vi "Cell12_PS_Control_Remote.vi"() -> ()   [LabVIEW 2021]
panel:
  in  "Slew Rate":dbl=1.0 format="%#_4g"
  out "error out 3":errorcluster
  in  "Setpoint [T]":dbl format="%#_4g"
  in  "stop":bool
  in  "port":u16=3376
  in  "error in (no error) 2":errorcluster
  in  "Data mac ip address":string="146.201.214.247"
  out "Field [T]":dbl=-17.9883723 format="%#_4g"
  # "[T/min]"
  # "Note\n(1) Exception of the firewall should be configured.\n(2) With some (not all) connection with PC's, it is successful only when the VI is first executed. If the VI is stopped (normally or by aborting), \nthe subsequent connection is only possible with a new port number."
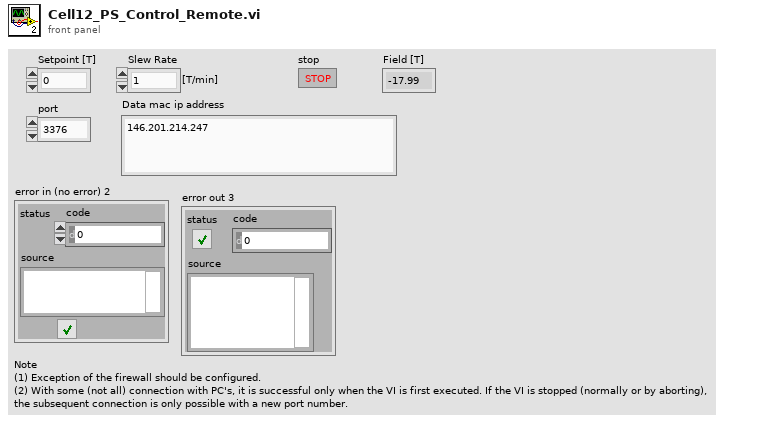
[diagram p1: front panel]
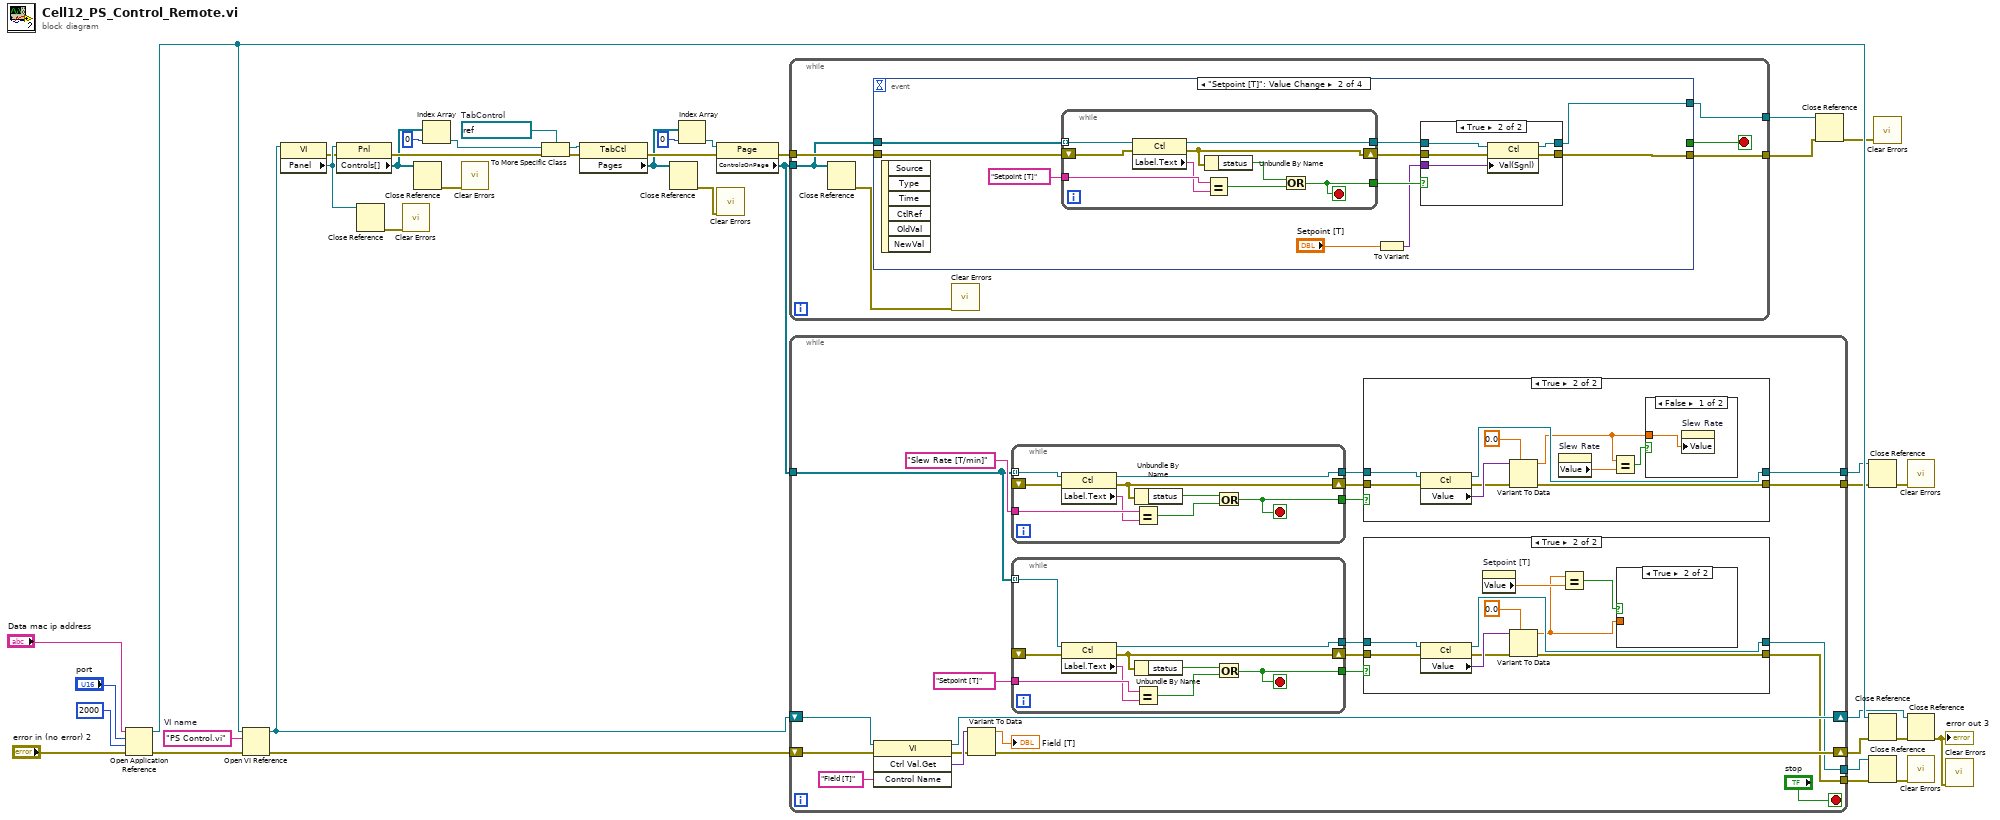
[diagram p0: block diagram]
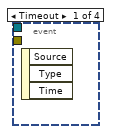
[diagram p2: hidden frame]
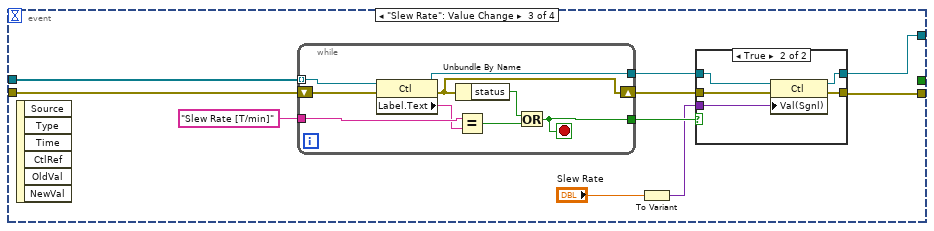
[diagram p4: hidden frame]
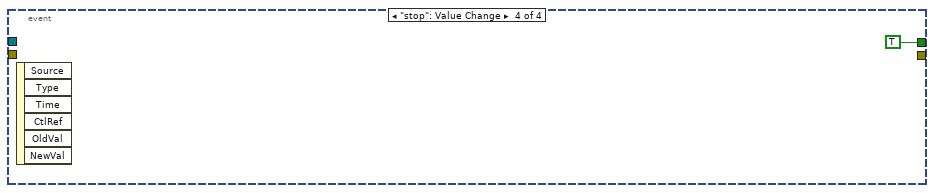
[diagram p6: hidden frame]
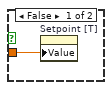
[diagram p8: hidden frame]
diagram:
  w13 = refnum<vi> refnum  # TabControl
  w32 = "PS Control.vi"  # VI name
  n1 = Open Application Reference(8:"error in (no error) 2", 9:2000 ("timeout ms (60000)"), 10:"port", 11:"Data mac ip address") -> (0:w39:errorcluster, 3:w34:refnum<vi>)
  n2 = Open VI Reference(application reference (local)=w34, vi path=w32, error in (no error)=w39) -> (vi reference=w29:refnum<vi>, error out=w28:errorcluster)  [unwired: 3 in]
  n3 = property class="VI"(reference=w29) -> (error out=w16:errorcluster, "Panel"=w19:refnum<vi>)  [unwired: 1 in, 1 out]
  n4 = property class="Pnl"(reference=w19, error in=w16) -> (error out=w25:errorcluster, "Controls[]"=w21:refnum<vi>[])  [unwired: 1 out]
  n5 = Close Reference(reference=w19) -> (error out=w15:errorcluster)  [unwired: 1 in]
  n6 = call <vilib>:"Clear Errors.vi"("error in (no error)"=w15) -> ()  [unwired: 5 in, 2 out]
  n7 = Close Reference(reference=w21) -> (error out=w20:errorcluster)  [unwired: 1 in]
  n8 = Index Array(array=w21, index=0) -> (element=w17:refnum<vi>)
  n9 = call <vilib>:"Clear Errors.vi"("error in (no error)"=w20) -> ()  [unwired: 5 in, 2 out]
  n10 = To More Specific Class(target class=w13, reference=w17, error in=w25) -> (specific class reference=w18:refnum<vi>, error out=w26:errorcluster)
  n11 = property class="TabCtl"(reference=w18, error in=w26) -> (error out=w27:errorcluster, "Pages"=w23:refnum<vi>[])  [unwired: 1 out]
  n12 = Close Reference(reference=w23) -> (error out=w22:errorcluster)  [unwired: 1 in]
  n13 = Index Array(array=w23, index=0) -> (element=w24:refnum<vi>)
  n14 = property class="Page"(reference=w24, error in=w27) -> (error out=w11:errorcluster, "ControlsOnPage"=w10:refnum<vi>[])  [unwired: 1 out]
  n15 = call <vilib>:"Clear Errors.vi"("error in (no error)"=w22) -> ()  [unwired: 5 in, 2 out]
  n16 = while {
    tunnel: w11 -> [w44]
    tunnel: w10 -> [w43]
    tunnel: [w42] -> w2
    tunnel: [w41] -> w1
    stop <- w46 stop-if-true
    n17 = Close Reference(reference=w43) -> (error out=w45:errorcluster)  [unwired: 1 in]
    n18 = event shown="[1] \"Setpoint [T]\": Value Change" {
      selector: _ -> [_ _ _ _]
      dyn-events: _ -> [_ _ _ _]
      timeout: _ -> [_ _ _ _]
      tunnel: [_ _ _ TRUE] -> w46
      tunnel: [_ w51 w76 _] -> w42
      tunnel: w44 -> [_ w50 w74 _]
      tunnel: w43 -> [_ w49 w75 _]
      tunnel: [_ w47 w73 _] -> w41
      event Timeout {
        n19 = event-data() -> ()  [unwired: 1 in, 3 out]
      }
      event "Setpoint [T]": Value Change {
        n20 = event-data() -> ()  [unwired: 1 in, 6 out]
        n21 = while {
          tunnel: w49 -> [w72] mode=indexing
          tunnel: "Setpoint [T]" ("Control Name") -> [w71]
          shift-right: [w68] -> w55
          shift-left: w50 -> [w70]
          tunnel: [w69] -> w48
          tunnel: [w65] -> w56
          stop <- w65 stop-if-true
          n22 = property class="Ctl"(reference=w72, error in=w70) -> (reference out=w69:refnum<vi>, error out=w68:errorcluster, "Label.Text"=w64:string)
          n23 = Unbundle By Name(w68) -> ("status"=w67:bool)
          n24 = Equal?(x=w71, y=w64) -> (x = y?=w66:bool)
          n25 = Or(x=w67, y=w66) -> (x .or. y?=w65:bool)
        }
        n26 = To Variant(anything="Setpoint [T]") -> (Variant=w52:variant)
        n27 = case shown="True" w56 {
          tunnel: w48 -> [w57 w62]
          tunnel: w55 -> [w58 w63]
          tunnel: [w58 w61] -> w47
          tunnel: [w57 w60] -> w51
          tunnel: w52 -> [_ w59]
          frame False {
          }
          frame True {
            n28 = property class="Ctl"(reference=w62, error in=w63, "Val(Sgnl)"=w59) -> (reference out=w60:refnum<vi>, error out=w61:errorcluster)
          }
        }
      }
      event "Slew Rate": Value Change {
        n29 = event-data() -> ()  [unwired: 1 in, 6 out]
        n30 = while {
          tunnel: w75 -> [w98] mode=indexing
          tunnel: "Slew Rate [T/min]" ("Control Name") -> [w97]
          shift-right: [w94] -> w80
          shift-left: w74 -> [w96]
          tunnel: [w95] -> w82
          tunnel: [w91] -> w81
          stop <- w91 stop-if-true
          n31 = property class="Ctl"(reference=w98, error in=w96) -> (reference out=w95:refnum<vi>, error out=w94:errorcluster, "Label.Text"=w90:string)
          n32 = Unbundle By Name(w94) -> ("status"=w93:bool)
          n33 = Equal?(x=w97, y=w90) -> (x = y?=w92:bool)
          n34 = Or(x=w93, y=w92) -> (x .or. y?=w91:bool)
        }
        n35 = To Variant(anything="Slew Rate") -> (Variant=w78:variant)
        n36 = case shown="True" w81 {
          tunnel: w82 -> [w83 w88]
          tunnel: w80 -> [w84 w89]
          tunnel: [w84 w87] -> w73
          tunnel: [w83 w86] -> w76
          tunnel: w78 -> [_ w85]
          frame False {
          }
          frame True {
            n37 = property class="Ctl"(reference=w88, error in=w89, "Val(Sgnl)"=w85) -> (reference out=w86:refnum<vi>, error out=w87:errorcluster)
          }
        }
      }
      event "stop": Value Change {
        n38 = event-data() -> ()  [unwired: 1 in, 6 out]
      }
    }
    n39 = call <vilib>:"Clear Errors.vi"("error in (no error)"=w45) -> ()  [unwired: 5 in, 2 out]
  }
  n40 = while {
    shift-right: [w119] -> w33
    shift-left: w29 -> [w114]
    shift-right: [w121] -> w36
    shift-left: w28 -> [w113]
    tunnel: w10 -> [w104]
    tunnel: [w103] -> w8
    tunnel: [w102] -> w7
    tunnel: [w101] -> w5
    tunnel: [w100] -> w4
    stop <- "stop" stop-if-true
    n41 = invoke class="VI" method="Ctrl Val.Get"(reference=w114, error in=w113, "Control Name"="Field [T]") -> (reference out=w119:refnum<vi>, error out=w117:errorcluster, "Get Control Value Variant"=w118:variant)  [unwired: 1 in, 1 out]
    n42 = Variant To Data(error in=w117, Variant=w118) -> (data=→"Field [T]":dbl, error out=w121:errorcluster)  [unwired: 1 in]
    n43 = while {
      tunnel: w104 -> [w165] mode=indexing
      tunnel: "Slew Rate [T/min]" ("Control Name") -> [w164]
      shift-right: [w161] -> w111
      shift-left: _ -> [w163]
      tunnel: [w162] -> w112
      tunnel: [w158] -> w110
      stop <- w158 stop-if-true
      n44 = property class="Ctl"(reference=w165, error in=w163) -> (reference out=w162:refnum<vi>, error out=w161:errorcluster, "Label.Text"=w157:string)
      n45 = Unbundle By Name(w161) -> ("status"=w160:bool)
      n46 = Equal?(x=w164, y=w157) -> (x = y?=w159:bool)
      n47 = Or(x=w160, y=w159) -> (x .or. y?=w158:bool)
    }
    n48 = while {
      tunnel: w104 -> [w143] mode=indexing
      tunnel: "Setpoint [T]" ("Control Name") -> [w142]
      shift-right: [w139] -> w108
      shift-left: _ -> [w141]
      tunnel: [w140] -> w109
      tunnel: [w136] -> w107
      stop <- w136 stop-if-true
      n49 = property class="Ctl"(reference=w143, error in=w141) -> (reference out=w140:refnum<vi>, error out=w139:errorcluster, "Label.Text"=w135:string)
      n50 = Unbundle By Name(w139) -> ("status"=w138:bool)
      n51 = Equal?(x=w142, y=w135) -> (x = y?=w137:bool)
      n52 = Or(x=w138, y=w137) -> (x .or. y?=w136:bool)
    }
    n53 = case shown="True" w110 {
      tunnel: w112 -> [w144 w155]
      tunnel: w111 -> [w145 w154]
      tunnel: [w145 w150] -> w100
      tunnel: [w144 w151] -> w101
      frame False {
      }
      frame True {
        n54 = property class="Ctl"(reference=w155, error in=w154) -> (reference out=w151:refnum<vi>, error out=w149:errorcluster, "Value"=w153:variant)
        n55 = Variant To Data(error in=w149, type=0.0, Variant=w153) -> (data=w146:dbl, error out=w150:errorcluster)
        n56 = property on="Slew Rate" class="DigNum (strict)"() -> ("Value"=w148:dbl)  [unwired: 2 in, 2 out]
        n57 = Equal?(x=w146, y=w148) -> (x = y?=w147:bool)
        n58 = case shown="False" w147 {
          tunnel: w146 -> [w156 _]
          frame False {
            n59 = property on="Slew Rate" class="DigNum (strict)"("Value"=w156) -> ()  [unwired: 2 in, 2 out]
          }
          frame True {
          }
        }
      }
    }
    n60 = case shown="True" w107 {
      tunnel: w109 -> [w122 w133]
      tunnel: w108 -> [w123 w132]
      tunnel: [w123 w128] -> w103
      tunnel: [w122 w129] -> w102
      frame False {
      }
      frame True {
        n61 = property class="Ctl"(reference=w133, error in=w132) -> (reference out=w129:refnum<vi>, error out=w127:errorcluster, "Value"=w131:variant)
        n62 = property on="Setpoint [T]" class="DigNum (strict)"() -> ("Value"=w126:dbl)  [unwired: 2 in, 2 out]
        n63 = Variant To Data(error in=w127, type=0.0, Variant=w131) -> (data=w125:dbl, error out=w128:errorcluster)
        n64 = Equal?(x=w125, y=w126) -> (x = y?=w124:bool)
        n65 = case shown="True" w124 {
          tunnel: w125 -> [w134 _]
          frame False {
            n66 = property on="Setpoint [T]" class="DigNum (strict)"("Value"=w134) -> ()  [unwired: 2 in, 2 out]
          }
          frame True {
          }
        }
      }
    }
  }
  n67 = Close Reference(reference=w2, error in (no error)=w1) -> (error out=w3:errorcluster)
  n68 = Close Reference(reference=w5, error in (no error)=w4) -> (error out=w6:errorcluster)
  n69 = Close Reference(reference=w34, error in (no error)=w36) -> (error out=w35:errorcluster)
  n70 = Close Reference(reference=w7, error in (no error)=w8) -> (error out=w9:errorcluster)
  n71 = call <vilib>:"Clear Errors.vi"("error in (no error)"=w3) -> ()  [unwired: 5 in, 2 out]
  n72 = call <vilib>:"Clear Errors.vi"("error in (no error)"=w6) -> ()  [unwired: 5 in, 2 out]
  n73 = Close Reference(reference=w33, error in (no error)=w35) -> (error out=w30:errorcluster)
  "error out 3" <- w30
  n74 = call <vilib>:"Clear Errors.vi"("error in (no error)"=w9) -> ()  [unwired: 5 in, 2 out]
  n75 = call <vilib>:"Clear Errors.vi"("error in (no error)"=w30) -> ()  [unwired: 5 in, 2 out]
